vi "set_eq_time.vi"(8 "error in (no error)":errorcluster, 10 "AOD equilibration time":dbl[unit], 11 "FPGAWrapperMH120124RAPS_PXI7813R in":refnum<class "FPGAWrapperMH120124RAPS_PXI7813R.lvclass">) -> (0 "error out":errorcluster, 3 "FPGAWrapperMH120124RAPS_PXI7813R out":refnum<class "FPGAWrapperMH120124RAPS_PXI7813R.lvclass">)   [LabVIEW 2010, in "FPGAWrapperMH120124RAPS_PXI7813R.lvclass"]
uses:
  FPGAWrapperMH120124RAPS_PXI7813R.lvclass
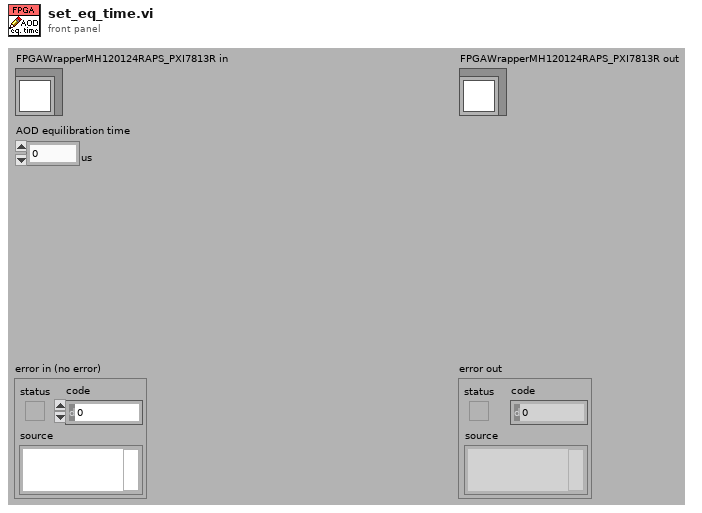
[diagram p1: front panel]
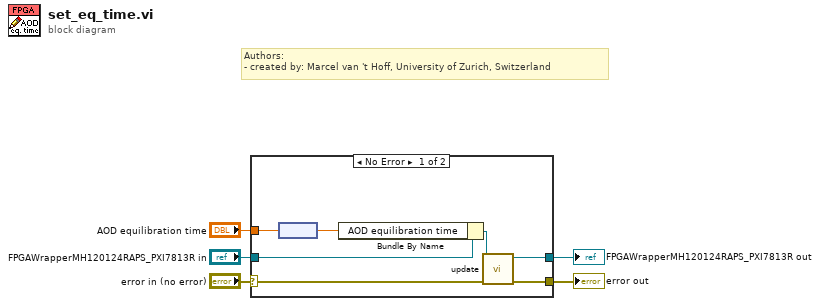
[diagram p0: block diagram]
diagram:
  # "Authors: \n- created by: Marcel van 't Hoff, University of Zurich, Switzerland"
  n1 = case shown="No Error" "error in (no error)" {
    selector: "error in (no error)" -> [w11 w13]
    tunnel: [w10 w13] -> w4
    tunnel: [w8 w14] -> w2
    tunnel: "FPGAWrapperMH120124RAPS_PXI7813R in" -> [w12 w14]
    tunnel: "AOD equilibration time" -> [w7 _]
    frame No Error {
      n2 = node(w7) -> (w6:dbl)
      n3 = Bundle By Name(cluster=w12, "AOD equilibration time"=w6) -> (w9:refnum<class "FPGAWrapperMH120124RAPS_PXI7813R.lvclass">)
      n4 = call-dynamic "update.vi"("error in (no error)"=w11, "FPGAWrapperMH120124RAPS_PXI7813R in"=w9) -> ("error out"=w10:errorcluster, "FPGAWrapperMH120124RAPS_PXI7813R out"=w8:refnum<class "FPGAWrapperMH120124RAPS_PXI7813R.lvclass">)  [unwired: 8 in]
    }
    frame Error {
    }
  }
  "error out" <- w4
  "FPGAWrapperMH120124RAPS_PXI7813R out" <- w2
